vi "Save Configuration.vi"(8 "error in (no error)":errorcluster, 10 "File path":path, 11 "Measure Object in":refnum<class "Measure Object.lvclass">) -> (0 "error out":errorcluster, 1 "Section out":string, 2 "File path out":path, 3 "Measure Object out":refnum<class "Measure Object.lvclass">)   [LabVIEW 2016, in "Measure Object.lvclass"]
uses:
  Measure Object.lvclass
  Measure Object.lvclass/Measure Object.ctl
  Measure Object Messages/Save Configuration Msg/Save Configuration Msg.lvclass/Save Configuration Msg.ctl
  <vilib>/ActorFramework/Message Enqueuer/Message Enqueuer.lvclass/Message Enqueuer.ctl
  Read Name.vi
  <vilib>/ActorFramework/Message Enqueuer/Enqueue.vi
  Measure Object Messages/Save Configuration Msg/Save Configuration Msg.lvclass
  D:/Program Files/National Instruments/LabVIEW 2016/vi.lib/ActorFramework/Message/Message.lvclass
  <vilib>/ActorFramework/Message Priority Queue/Priority Enqueue.vi
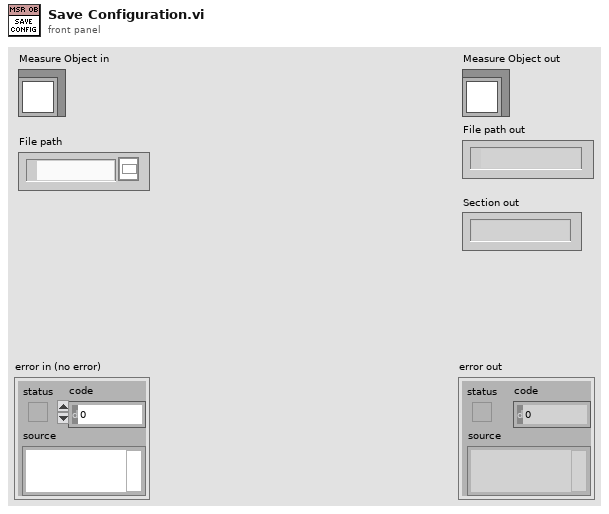
[diagram p1: front panel]
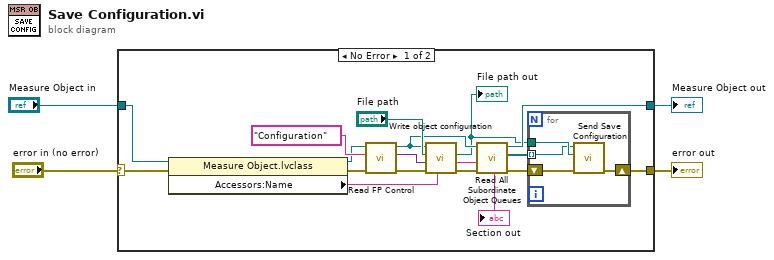
[diagram p0: block diagram]
diagram:
  n1 = case shown="No Error" "error in (no error)" {
    selector: "error in (no error)" -> [w16 w27]
    tunnel: [w9 w27] -> w3
    tunnel: [w10 w26] -> w1
    tunnel: "Measure Object in" -> [w15 w26]
    frame No Error {
      n2 = property class="Measure Object.lvclass"(reference=w15, error in=w16) -> (reference out=w14:refnum<class "Measure Object.lvclass">, error out=w17:errorcluster, "Accessors:Name"=w20:string)
      n3 = call-dynamic "Read FP Control.vi"("error in (no error)"=w17, "Control Name"="Configuration", "Measure Object in"=w14) -> ("error out"=w8:errorcluster, "Control Value"=w19:variant, "Measure Object out"=w11:refnum<class "Measure Object.lvclass">)  [unwired: 5 in, 1 out]
      n4 = call "Write object configuration.vi"("Object name"=w20, "Error In"=w8, "Configuration"=w19, "File path"="File path", "object"=w11) -> ("Error Out"=w7:errorcluster, "Section out"=→"Section out":string, "File path out"=w6:path)  [unwired: 4 in]
      "File path out" <- w6
      n5 = call-dynamic "Read All Subordinate Object Queues.vi"("error in (no error)"=w7, "Measure Object in"=w11) -> ("error out"=w12:errorcluster, "Object enqueuers"=w13:refnum<class "Message Enqueuer.lvclass">[], "Measure Object out"=w10:refnum<class "Measure Object.lvclass">)  [unwired: 6 in, 1 out]
      n6 = for {
        tunnel: w6 -> [w25]
        tunnel: w13 -> [w24] mode=indexing
        shift-right: [w23] -> w9
        shift-left: w12 -> [w22]
        n7 = call "Send Save Configuration.vi"("error in (no error)"=w22, "File path"=w25, "Message Enqueuer"=w24) -> ("error out"=w23:errorcluster)  [unwired: 7 in, 1 out]
      }
    }
    frame Error {
    }
  }
  "error out" <- w3
  "Measure Object out" <- w1
